vi "DrawPlot.vi"() -> ()   [LabVIEW 2017]
panel:
  out "Graph":cluster{i32[], dbl[]}(graph)
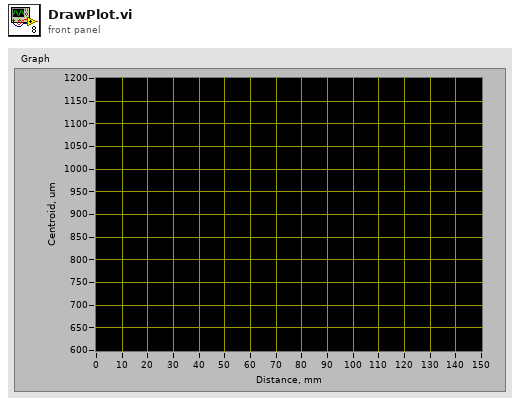
[diagram p1: front panel]
types:
  T1 = cluster{"Centroid of max, um":dbl, "Centroid of width, um":dbl, "Width, um":dbl, "Width, px":i32, "Beam Angle, mrad":dbl, "Divergence, mrad":dbl}[]
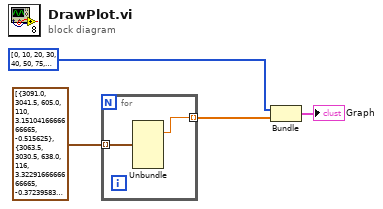
[diagram p0: block diagram]
diagram:
  n1 = for {
    tunnel: T1 [{"Centroid of max, um"=3091.0, "Centroid of width, um"=3041.5, "Width, um"=605.0, "Width, px"=110, "Beam Angle, mrad"=3.1510416666666665, "Divergence, mrad"=-0.515625}, {"Centroid of max, um"=3063.5, "Centroid of width, um"=3030.5, "Width, um"=638.0, "Width, px"=116, "Beam Angle, mrad"=3.3229166666666665, "Divergence, mrad"=-0.37239583333333337}, {"Centroid of max, um"=3052.5, "Centroid of width, um"=3011.25, "Width, um"=654.5, "Width, px"=119, "Beam Angle, mrad"=3.408854166666667, "Divergence, mrad"=-0.31510416666666663}, {"Centroid of max, um"=3047.0, "Centroid of width, um"=3011.25, "Width, um"=698.5, "Width, px"=127, "Beam Angle, mrad"=3.6380208333333335, "Divergence, mrad"=-0.2864583333333333}, {"Centroid of max, um"=3074.5, "Centroid of width, um"=2997.5, "Width, um"=726.0, "Width, px"=132, "Beam Angle, mrad"=3.78125, "Divergence, mrad"=-0.4296875}, {"Centroid of max, um"=3074.5, "Centroid of width, um"=2989.25, "Width, um"=764.5, "Width, px"=139, "Beam Angle, mrad"=3.9817708333333335, "Divergence, mrad"=-0.4296875}, {"Centroid of max, um"=3052.5, "Centroid of width, um"=2953.5, "Width, um"=891.0, "Width, px"=162, "Beam Angle, mrad"=4.640625, "Divergence, mrad"=-0.31510416666666663}, {"Centroid of max, um"=3019.5, "Centroid of width, um"=2923.25, "Width, um"=1039.5, "Width, px"=189, "Beam Angle, mrad"=5.4140625, "Divergence, mrad"=-0.14322916666666666}, {"Centroid of max, um"=2964.5, "Centroid of width, um"=2901.25, "Width, um"=1182.5, "Width, px"=215, "Beam Angle, mrad"=6.158854166666667, "Divergence, mrad"=0.14322916666666666}] ("Fast Axis Array") -> [w6] mode=indexing
    tunnel: [w5] -> w1 mode=indexing
    n2 = Unbundle(w6) -> ("Centroid of width, um"=w5:dbl)  [unwired: 5 out]
  }
  n3 = Bundle("Index"=i32[] [0, 10, 20, 30, 40, 50, 75, 100, 150], w1) -> (→"Graph":cluster{"Index":i32[], dbl[]})  [unwired: 1 in]
